vi "Read_FPGA.vi"() -> ()   [LabVIEW 2019]
uses:
  <vilib>/Platform/TimedLoop/XDataNode/timing_clust.ctl
  <vilib>/Platform/TimedLoop/XDataNode/nitl_modes.ctl
  <vilib>/Platform/TimedLoop/XDataNode/wakeup.ctl
  <vilib>/FPGAPlugInAG/myRIO-1900/niLvFpga_Open_myRIO-1900.vi
  <vilib>/rvi/interface/common/dynamic/niFpgaDynamicAddResources.vi
  <vilib>/rvi/interface/common/niFpgaWaitOnOcc.vi
  <vilib>/Utility/error.llb/Error Cluster From Error Code.vi
  <vilib>/FPGAPlugInAG/Dynamic/niLvFpga_Run_Dynamic.vi
  <vilib>/rvi/errors/niLvFpgaAdjustHostInterfaceError.vi
  <vilib>/FPGAPlugInAG/Dynamic/niLvFpga_Close_Dynamic.vi
  <vilib>/rvi/interface/nirviOpenFPGA/nirviOpenFPGA.xnode
  FPGA Bitfiles/FPGAp_FPGATarget_FPGA1_1pLoeQXMOaA.lvbitx
  FPGA_1.vi
  <vilib>/rvi/interface/nirviMethod/nirviMethod.xnode
  <vilib>/platform/TimedLoop/XDataNode/XDataNode.xnode
  <vilib>/rvi/interface/nirviCloseFPGA/nirviCloseFPGA.xnode
  <vilib>/rvi/errors/niLvFpgaMergeErrorWithErrorCode.vi
  <vilib>/Platform/TimedLoop/XDataNode/XDNodeRunTimeDep.lvlib
  <vilib>/FPGAPlugInAG/Dynamic/niLvFpga_ReadFifo_Dynamic.vi
  <vilib>/FPGAPlugInAG/Dynamic/niLvFpga_ConfigureFifo_Dynamic.vi
  <vilib>/FPGAPlugInAG/Dynamic/niLvFpga_StartFifo_Dynamic.vi
  <vilib>/FPGAPlugInAG/Dynamic/niLvFpga_StopFifo_Dynamic.vi
panel:
  in  "file path 3":path
  in  "file path 2":path
  out "error out":errorcluster
  out "Data 3":u16[](graph)
  out "data 3":u16[](array[numeric])
  out "data 1":u16[](array[numeric])
  out "data 2":u16[](array[numeric])
  out "Data 1":u16[](graph)
  in  "file path":path
  in  "stop":bool
  out "Data 2":u16[](graph)
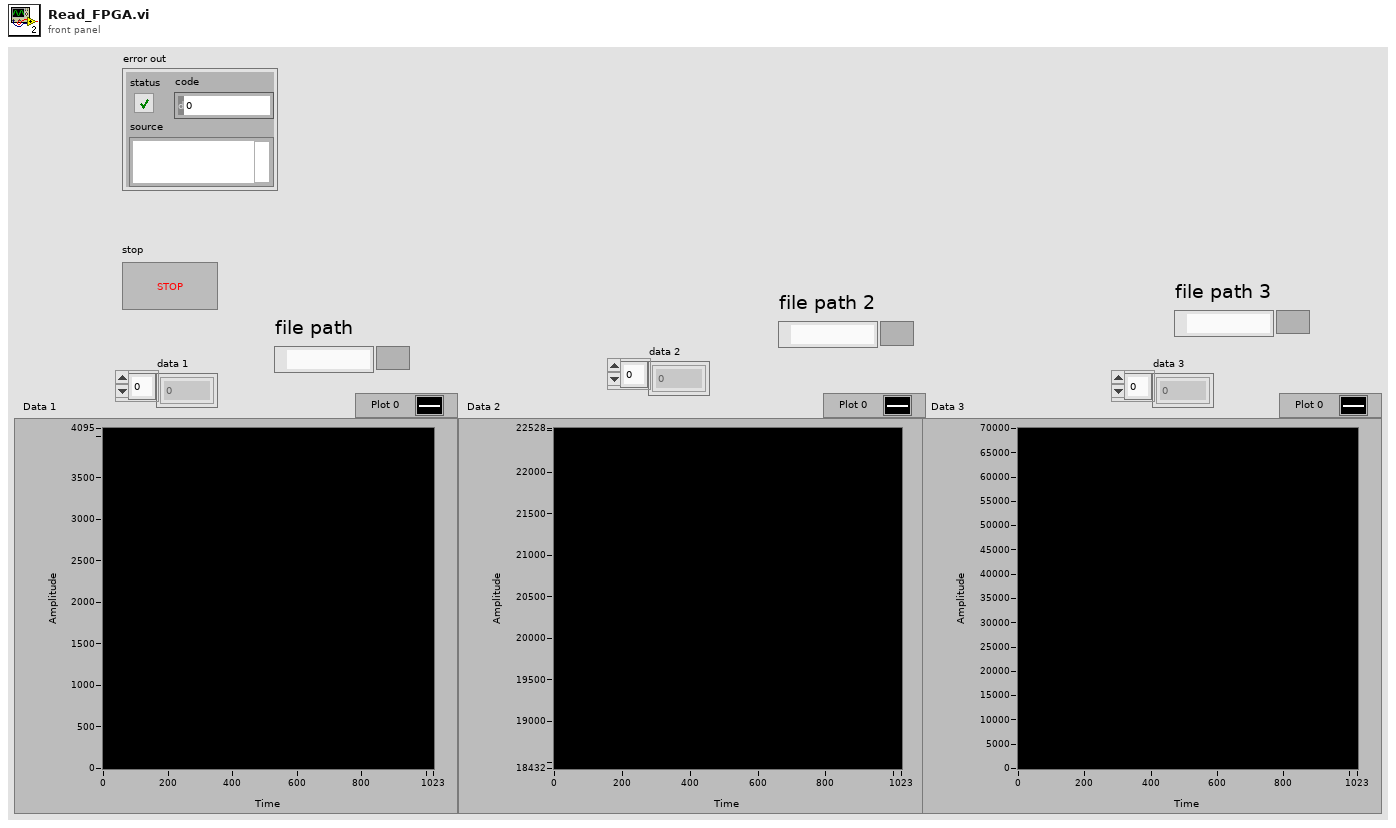
[diagram p1: front panel]
types:
  T1 = enum16{"open", "open or create", "create or replace", "create", "open (read-only)"}
  T2 = typedef "XDNodeRunTimeDep.lvlib/timing_clust.ctl" = cluster{"Expected End [f-1]":u64, "Actual End [f-1]":u64, "Finished Late? [f-1]":bool, "Expected End [i-1]":u64, "Actual End [i-1]":u64, "Finished Late? [i-1]":bool, "Expected Start [i]":u64, "Actual Start [i]":u64, "Expected Start [f]":u64, "Actual Start [f]":u64, "Source Name":string, "Structure Name":string, "Period":i64, "Deadline":i64, "Offset":i64, "Start":i64, "Priority":i32, "Timeout":i32, "Mode":T3, "Wakeup Reason":T4, "Error":errorcluster, "Source Type":string, "Secondary Source Type":string, "Global End Time":u64, "Global Start Time":u64, "Frame Duration":u64, "Iteration Duration":u64, "Assigned CPU":i32, "I/O Scan Engine Mode":u32}
  T3 = typedef "XDNodeRunTimeDep.lvlib/nitl_modes.ctl" = enum32{"No Change", "Process missed periods, maintain original phase", "Discard missed periods, maintain original phase", "Process missed periods, ignore original phase", "Discard missed periods, ignore original phase"}
  T4 = typedef "XDNodeRunTimeDep.lvlib/wakeup.ctl" = enum32{"Normal", "Aborted", "Asynchronous wakeup", "Timing source error", "Timed loop error", "Timeout"}
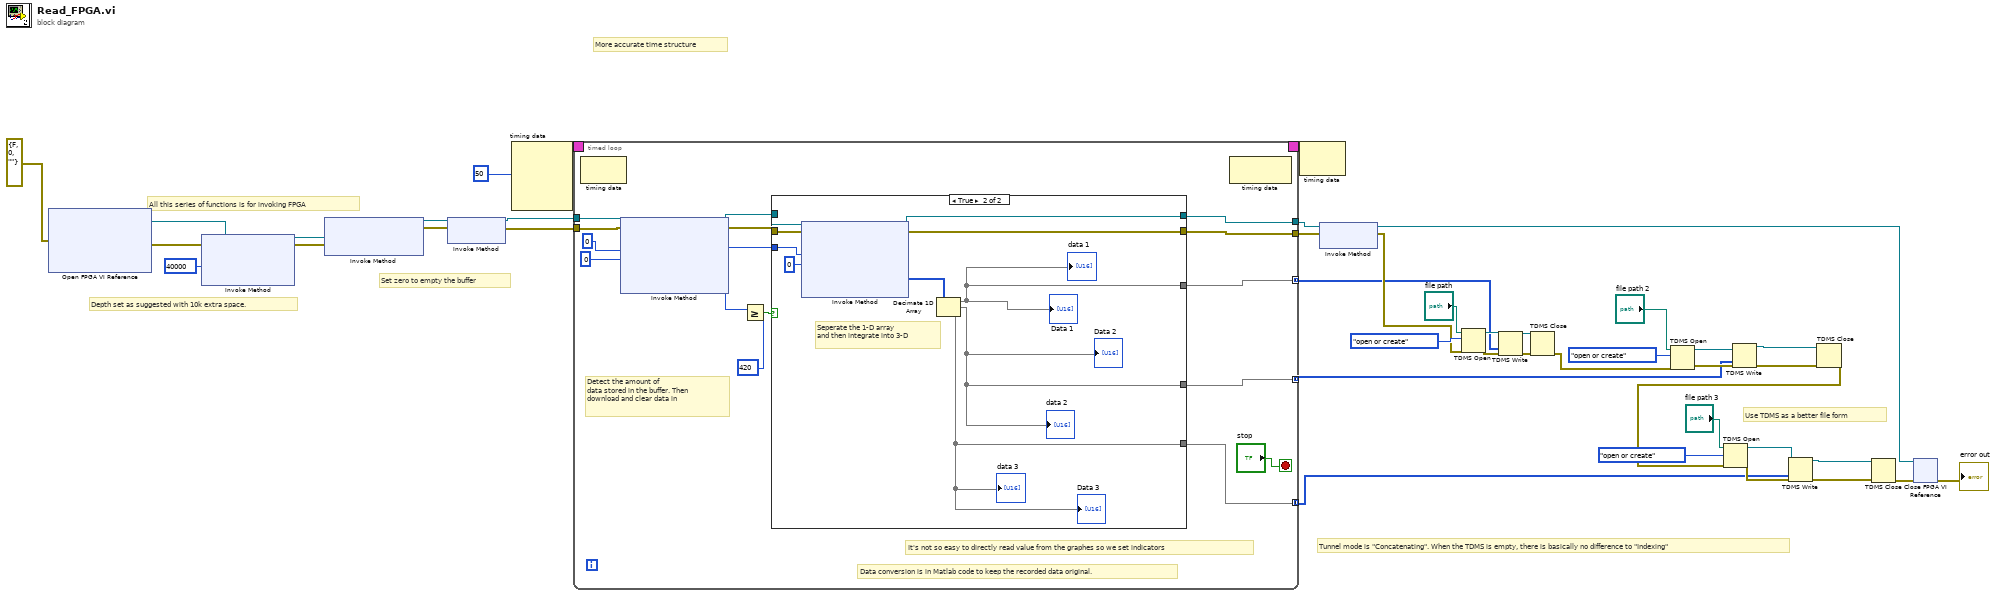
[diagram p0: block diagram]
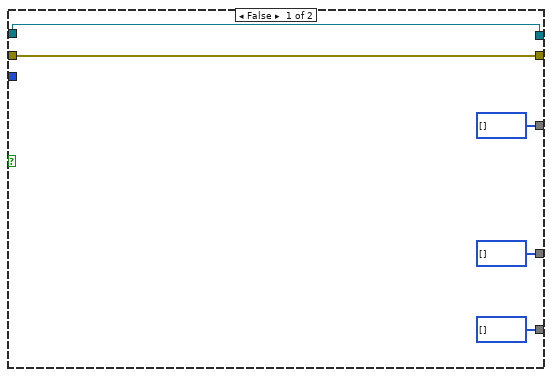
[diagram p2: hidden frame]
diagram:
  # "Use TDMS as a better file form"
  # "Tunnel mode is \"Concatenating\". When the TDMS is empty, there is basically no difference to \"Indexing\""
  # "Set zero to empty the buffer"
  # "More accurate time structure"
  # "All this series of functions is for invoking FPGA"
  # "Depth set as suggested with 10k extra space."
  n1 = xnode "Open FPGA VI Reference"("error in"=errorcluster {"status"=FALSE, "code"=0, "source"=""} ("error constant")) -> ("FPGA VI Reference Out"=w42:refnum<k20>, "error out"=w41:errorcluster)  [unwired: 1 in]
  n2 = xnode "Invoke Method"("FPGA VI Reference In"=w42, "error in"=w41, "Requested Depth"=u32 40000) -> ("FPGA VI Reference Out"=w40:refnum<k20>, "error out"=w39:errorcluster)  [unwired: 1 out]
  n3 = xnode "Invoke Method"("FPGA VI Reference In"=w40, "error in"=w39) -> ("FPGA VI Reference Out"=w38:refnum<k20>, "error out"=w37:errorcluster)  [unwired: 1 in]
  n4 = xnode "Invoke Method"("FPGA VI Reference In"=w38, "error in"=w37) -> ("FPGA VI Reference Out"=w36:refnum<k20>, "error out"=w35:errorcluster)
  n5 = node-c288(i64 50 ("Period")) -> (w31:T2)  [unwired: 3 in]
  n6 = timed-loop {
    tunnel: w36 -> [w54]
    tunnel: w35 -> [w53]
    timing: w31 -> [_]
    timing-out: [_] -> w30
    tunnel: [w49] -> w20
    tunnel: [w48] -> w19
    tunnel: [w45] -> w6 mode=concatenating
    tunnel: [w44] -> w2 mode=concatenating
    tunnel: [w43] -> w1 mode=concatenating
    stop <- "stop" stop-if-true
    # "Data conversion is in Matlab code to keep the recorded data original."
    # "It's not so easy to directly read value from the graphes so we set indicators"
    # "Detect the amount of \ndata stored in the buffer. Then \ndownload and clear data in"
    n7 = node-c288() -> ()  [unwired: 1 in, 1 out]
    n8 = xnode "Invoke Method"("FPGA VI Reference In"=w54, "error in"=w53, "Number of Elements"=u32 0, "Timeout (ms)"=0) -> ("FPGA VI Reference Out"=w47:refnum<k20>, "error out"=w46:errorcluster, "Elements Remaining"=w50:u32)  [unwired: 1 out]
    n9 = Greater Or Equal?(x=w50, y=u32 420) -> (x >= y?=w51:bool)
    n10 = case shown="True" w51 {
      tunnel: w50 -> [_ w72]
      tunnel: [w62 w71] -> w49
      tunnel: [w61 w70] -> w48
      tunnel: w47 -> [w61 w69]
      tunnel: w46 -> [w62 w68]
      tunnel: [u16[] [] w65] -> w45
      tunnel: [u16[] [] w64] -> w44
      tunnel: [u16[] [] w63] -> w43
      frame False {
      }
      frame True {
        # "Seperate the 1-D array\nand then integrate into 3-D"
        n11 = xnode "Invoke Method"("FPGA VI Reference In"=w69, "error in"=w68, "Number of Elements"=w72, "Timeout (ms)"=0) -> ("FPGA VI Reference Out"=w70:refnum<k20>, "error out"=w71:errorcluster, "Data"=w67:u16[])  [unwired: 1 out]
        n12 = Decimate 1D Array "Decimate 1D Array"(w67) -> (w65:u16[], w64:u16[], w63:u16[])
        "Data 2" <- w64
        "Data 1" <- w65
        "data 2" <- w64
        "data 1" <- w65
        "data 3" <- w63
        "Data 3" <- w63
      }
    }
    n13 = node-c288() -> ()  [unwired: 1 in, 1 out]
  }
  n14 = node-c288(w30) -> ()  [unwired: 1 out]
  n15 = xnode "Invoke Method"("FPGA VI Reference In"=w19, "error in"=w20) -> ("FPGA VI Reference Out"=w34:refnum<k20>, "error out"=w22:errorcluster)
  n16 = TDMS Open(8:w22, 10:T1."open or create" ("operation (0:open)"), 11:"file path") -> (0:w23:errorcluster, 3:w24:refnum<k34>)  [unwired: 4 in]
  n17 = TDMS Write(0:w24, 9:w6, 11:w23) -> (4:w25:refnum<k34>, 15:w26:errorcluster)  [unwired: 3 in, 2 out]
  n18 = TDMS Close(8:w26, 11:w25) -> (0:w5:errorcluster)  [unwired: 1 out]
  n19 = TDMS Open(8:w5, 10:T1."open or create" ("operation (0:open)"), 11:"file path 2") -> (0:w18:errorcluster, 3:w17:refnum<k34>)  [unwired: 4 in]
  n20 = TDMS Write(0:w17, 9:w2, 11:w18) -> (4:w16:refnum<k34>, 15:w15:errorcluster)  [unwired: 3 in, 2 out]
  n21 = TDMS Close(8:w15, 11:w16) -> (0:w4:errorcluster)  [unwired: 1 out]
  n22 = TDMS Open(8:w4, 10:T1."open or create" ("operation (0:open)"), 11:"file path 3") -> (0:w7:errorcluster, 3:w8:refnum<k34>)  [unwired: 4 in]
  n23 = TDMS Write(0:w8, 9:w1, 11:w7) -> (4:w9:refnum<k34>, 15:w10:errorcluster)  [unwired: 3 in, 2 out]
  n24 = TDMS Close(8:w10, 11:w9) -> (0:w3:errorcluster)  [unwired: 1 out]
  n25 = xnode "Close FPGA VI Reference"("FPGA VI Reference In"=w34, "error in"=w3) -> ("error out"=→"error out":errorcluster)
